vi "Polarmeter_param.vi"() -> ()   [LabVIEW 2018]
panel:
  in  "触发电压":u64(ring)=200 items=["200mv"=200, "20mv"=20, "2mv"=2]
  in  "时间范围":u64(ring)=100000 items=["100ms"=1000000000, "10ms"=100000000, "1ms"=10000000, "100us"=1000000, "10us"=100000, "1us"=10000, "100ns"=1000, "10ns"=100, "1ns"=10, "100ps"=1]
  in  "电压范围":u64(ring)=10 items=["1 V"=1000000, "100mv"=100000, "10mv"=10000, "1mv"=1000, "100uv"=100, "10uv"=10]
  in  "示波器通道":T1(ring)
  # "偏振仪\n参数"
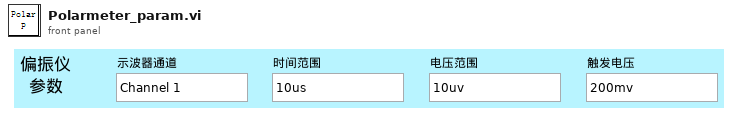
[diagram p1: front panel]
types:
  T1 = enum16{"Channel 1", "Channel 2", "Channel 3", "Channel 4"}
  T2 = typedef "IMAQ Image.ctl" = refnum<image>
  T3 = cluster{"示波器":cluster{"Channel (0:Channel 1)":enum16{"Channel 1", "Channel 2", "Channel 3", "Channel 4"}, "电压范围":dbl, "触发电压":dbl, "时间范围":dbl, " 示波器VISA":refnum<visa-resource-name>, "时间范围 标签":u64, "电压范围 标签":u64, "触发电压 标签":u64}, "光谱仪":cluster{"Channel (0:Channel 1)":enum16{"Channel 1", "Channel 2", "Channel 3", "Channel 4"}, "电压范围":u64, "触发电压":u64, "时间范围":u64}, " 近场相机":cluster{"曝光时间":i32, "模拟增益":i32, "控制套接字":i32, "IP 地址":string, " 采集套接字":i32, "  版本号":i32, "ImageData":T2, "  增益最大":i32, "  增益最小":i32, " 曝光最大":i32, " 曝光最小":i32, " 帧速":i32, " 同步切换":i32, "  曝光缩放":i32}, " 偏振仪":cluster{"电压范围":u64, "触发电压":u64, "时间范围":u64, "波长范围":enum16{"可见光 400-700nm", "近红外 700-1100nm"}, "可见光偏振测量仪VISA":refnum<visa-resource-name>, "近红外偏振测量仪VISA":refnum<visa-resource-name>}, " 功率计":cluster{"通道":enum16{"Channel 1", "Channel 2"}, "工作波长":u32, "单位":u64, "时间范围":u64, "IP地址":string, "端口":u32}, "能量计":cluster{"通道":enum16{"Channel 1", "Channel 2"}, "工作波长":u32, "单位":u64, "时间范围":u64, "IP地址":string, "端口":u32, "能量计量程":enum16{"200uJ", "20uJ", "2uJ", "200nJ"}}, "电机":cluster{"Channel (0:Channel 1)":enum16{"Channel 1", "Channel 2", "Channel 3", "Channel 4"}, "电压范围":u64, "触发电压":u64, "时间范围":u64}, " 远场相机":cluster{"曝光时间":i32, "模拟增益":i32, "控制套接字":i32, "IP 地址":string, " 采集套接字":i32, "  版本号":i32, "ImageData":T2, "  增益最大":i32, "  增益最小":i32, " 曝光最大":i32, " 曝光最小":i32, " 帧速":i32, " 同步切换":i32, "  曝光缩放":i32}}
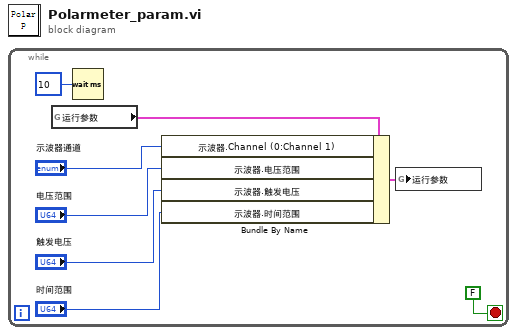
[diagram p0: block diagram]
diagram:
  n1 = while {
    stop <- FALSE stop-if-true
    n2 = global read "参数.vi" "运行参数"() -> (w6:T3)
    n3 = Wait (ms)(milliseconds to wait=u32 10 ("等待时间（毫秒）")) -> ()  [unwired: 1 out]
    n4 = Bundle By Name(cluster=w6, "示波器.Channel (0:Channel 1)"="示波器通道", "示波器.电压范围"="电压范围", "示波器.触发电压"="触发电压", "示波器.时间范围"="时间范围") -> (w3:T3)
    n5 = global write "参数.vi" "运行参数"(w3) -> ()
  }
